vi "MotorsGlobal.vi"() -> ()   [LabVIEW 2019]
uses:
  TurretMode.ctl
panel:
  in  "LL In Range?":bool
  in  "FlywheelSetpoint":dbl
  in  "IntakeRightIR":bool
  in  "IntakeLeftIR":bool
  in  "ConveyorIR":bool
  in  "IntakePiston":bool
  in  "Led0":bool
  in  "Led1":bool
  in  "EnableFlyWheel":bool
  in  "ResetYaw":bool
  out "Yaw":dbl
  in  "CompressorOn":bool
  in  "PTOSolenoid":bool
  in  "Climber On?":bool
  in  "ClimberOutput":dbl
  in  "Reset Encoder":bool
  out "TurretEncoder":dbl
  out "LL Mode":dbl
  out "LL LED Status":dbl
  in  "LL Valid Target?":bool
  out "LeftEncoder":dbl
  out "RightEncoder":dbl
  out "Amount of balls":dbl
  in  "TurretMode":T1
  in  "AutoTurret":bool
  in  "RollerOutput":dbl
  in  "ClimberSolenoid":bool
  in  "HoodSolenoid":bool
  in  "IntakeSolenoid":bool
  out "LimelightY":dbl
  out "LimelightX":dbl
  out "FlyWheelRate":dbl
  out "FlyWheelEncoder":dbl
  in  "ConveyorRightOutput":dbl
  in  "ConveyorLeftOutput":dbl
  in  "ConveyorMidOutput":dbl
  in  "IntakeOutput":dbl
  in  "TurretOutput":dbl
  in  "FlywheelOutput":dbl
  # "0 - Pipeline\n1 - Off\n2 - Blink\n3 - On"
  # "0 - Vision Processing\n1 - DS Camera"
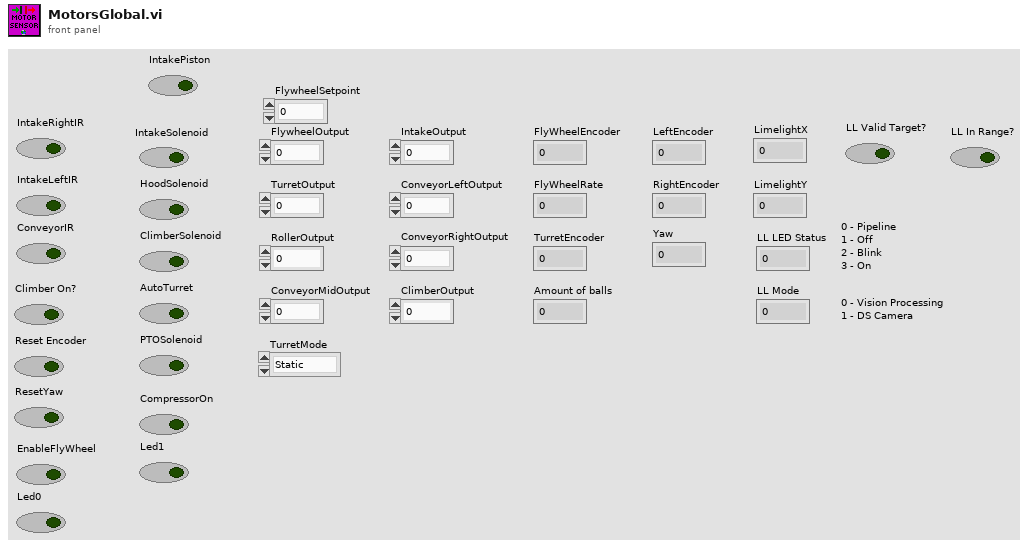
[diagram p1: front panel]
types:
  T1 = typedef "TurretMode.ctl" = enum16{"Static", "Manual", "Automatic"}
diagram:
